vi "WSP2_PartNumberRef.vi"(1 "BCTYPE":i8, 2 "SerialNumber":string) -> (0 "AssemblyPartNumber":string)   [LabVIEW 2017]
uses:
  C:/ClubCar EOL/WSConnector/WSConnector.dll
  WSConnector/WSConnector.dll
panel:
  out "Cimp_AssemblyPartNumber":string
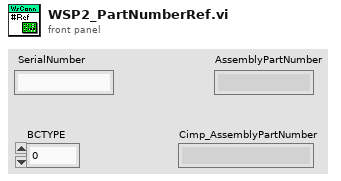
[diagram p1: front panel]
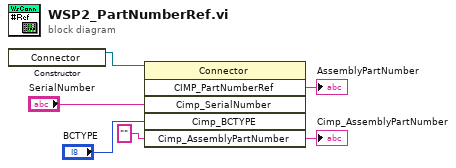
[diagram p0: block diagram]
diagram:
  n1 = constructor class="Connector"() -> (reference out=w6:refnum<k24>)  [unwired: 3 in, 2 out]
  n2 = invoke class="Connector" method="CIMP_PartNumberRef"(reference=w6, "Cimp_SerialNumber"="SerialNumber", "Cimp_BCTYPE"="BCTYPE", "Cimp_AssemblyPartNumber"="") -> ("CIMP_PartNumberRef"=→"AssemblyPartNumber":string, "Cimp_AssemblyPartNumber"=→"Cimp_AssemblyPartNumber":string)  [unwired: 2 in, 4 out]
